vi "meth.PushLVData.vi"(0 "class.GLue in":refnum<class "class.GLue.lvclass">, 7 "variant in":variant, 11 "error in (no error)":errorcluster) -> (4 "class.GLue out":refnum<class "class.GLue.lvclass">, 8 "NumPushed":i32, 15 "error out":errorcluster)   [LabVIEW 2014, in "GLue.lvlib" / "class.GLue.lvclass"]
uses:
  class.GLue.lvclass
  class.GLue.lvclass/class.GLue.ctl
  vi.HeaderFromTD.vi
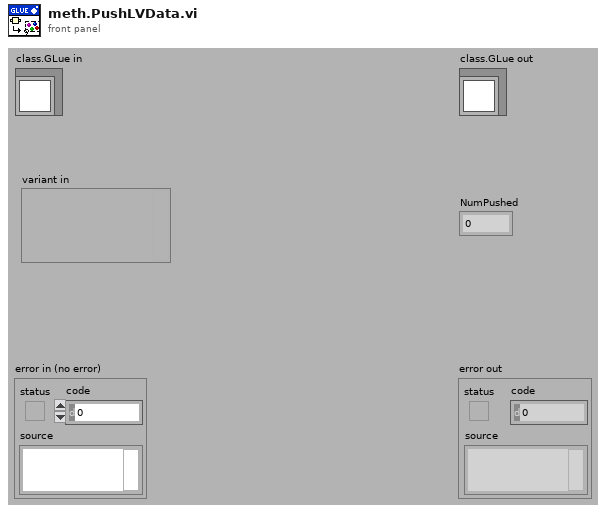
[diagram p1: front panel]
types:
  T1 = enum8{"<Null>", "I8", "I16", "I32", "I64", "U8", "U16", "U32", "U64", "SGL", "DBL", "EXT", "CSG", "CDB", "CXT", "0x0F", "0x10", "0x11", "0x12", "0x13", "0x14", "Enum U8", "Enum U16", "Enum U32", "Enum U64", "SGL PQ", "DBL PQ", "EXT PQ", "CSG PQ", "CDB PQ", "CXT PQ", "0x1F", "0x20", "Boolean", "0x22", "0x23", "0x24", "0x25", "0x26", "0x27", "0x28", "0x29", "0x2A", "0x2B", "0x2C", "0x2D", "0x2E", "0x2F", "String", "0x31", "Path", "Pict", "0x34", "0x35", "0x36", "DAQ", "0x38", "0x39", "0x3A", "0x3B", "0x3C", "0x3D", "0x3E", "0x3F", "Array", "0x41", "0x42", "0x43", "0x44", "0x45", "0x46", "0x47", "0x48", "0x49", "0x4A", "0x4B", "0x4C", "0x4D", "0x4E", "0x4F", "Cluster", "0x51", "0x52", "Variant", "Waveform", "0x55", "0x56", "0x57", "0x58", "0x59", "0x5A", "0x5B", "0x5C", "0x5D", "0x5E", "0x5F", "0x60", "0x61", "0x62", "0x63", "0x64", "0x65", "0x66", "0x67", "0x68", "0x69", "0x6A", "0x6B", "0x6C", "0x6D", "0x6E", "0x6F", "Refnum"}
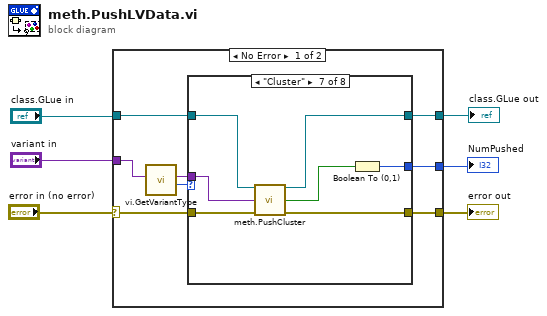
[diagram p0: block diagram]
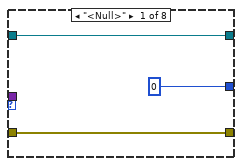
[diagram p2: hidden frame]
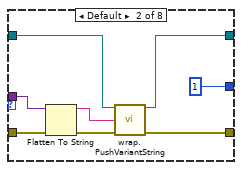
[diagram p3: hidden frame]
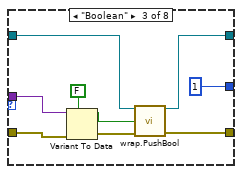
[diagram p4: hidden frame]
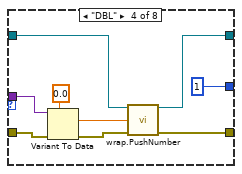
[diagram p5: hidden frame]
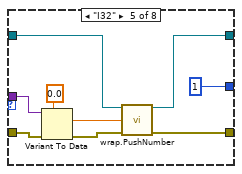
[diagram p6: hidden frame]
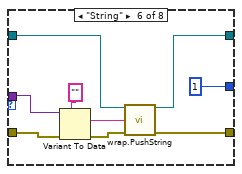
[diagram p7: hidden frame]
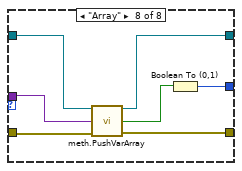
[diagram p8: hidden frame]
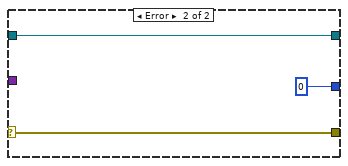
[diagram p9: hidden frame]
diagram:
  n1 = case shown="No Error" "error in (no error)" {
    selector: "error in (no error)" -> [w12 w78]
    tunnel: [w14 w78] -> w5
    tunnel: [w13 w77] -> w2
    tunnel: "class.GLue in" -> [w9 w77]
    tunnel: "variant in" -> [w8 _]
    tunnel: [w7 0] -> w1
    frame No Error {
      n2 = call "vi.GetVariantType.vi"("variant in"=w8) -> ("type"=w10:T1, "variant out"=w11:variant)  [unwired: 9 in]
      n3 = case shown="\"Cluster\"" w10 {
        tunnel: w11 -> [_ w19 w28 w37 w46 w55 w66 w69]
        tunnel: w9 -> [w16 w24 w29 w38 w47 w56 w68 w74]
        tunnel: w12 -> [w17 w22 w31 w40 w49 w58 w67 w75]
        tunnel: [w17 w25 w30 w39 w48 w57 w64 w72] -> w14
        tunnel: [w16 w23 w27 w36 w45 w54 w65 w73] -> w13
        tunnel: [0 1 1 1 1 1 w62 w71] -> w7
        frame "<Null>" {
        }
        frame Default {
          n4 = Flatten To String(anything=w19, error in (no error)=w22) -> (data string=w20:string, error out=w21:errorcluster)  [unwired: 2 in, 1 out]
          n5 = call "wrap.PushVariantString.vi"("class.GLue in"=w24, "VariantString"=w20, "error in (no error)"=w21) -> ("class.GLue out"=w23:refnum<class "class.GLue.lvclass">, "error out"=w25:errorcluster)  [unwired: 11 in]
        }
        frame "Boolean" {
          n6 = Variant To Data(error in=w31, type=FALSE, Variant=w28) -> (data=w34:bool, error out=w33:errorcluster)
          n7 = call "wrap.PushBool.vi"("class.GLue in"=w29, "Boolean"=w34, "error in (no error)"=w33) -> ("class.GLue out"=w27:refnum<class "class.GLue.lvclass">, "error out"=w30:errorcluster)  [unwired: 11 in]
        }
        frame "DBL" {
          n8 = Variant To Data(error in=w40, type=0.0, Variant=w37) -> (data=w41:dbl, error out=w42:errorcluster)
          n9 = call "wrap.PushNumber.vi"("class.GLue in"=w38, "Numeric"=w41, "error in (no error)"=w42) -> ("class.GLue out"=w36:refnum<class "class.GLue.lvclass">, "error out"=w39:errorcluster)  [unwired: 11 in]
        }
        frame "I32" {
          n10 = Variant To Data(error in=w49, type=0.0, Variant=w46) -> (data=w50:dbl, error out=w51:errorcluster)
          n11 = call "wrap.PushNumber.vi"("class.GLue in"=w47, "Numeric"=w50, "error in (no error)"=w51) -> ("class.GLue out"=w45:refnum<class "class.GLue.lvclass">, "error out"=w48:errorcluster)  [unwired: 11 in]
        }
        frame "String" {
          n12 = Variant To Data(error in=w58, type="", Variant=w55) -> (data=w61:string, error out=w60:errorcluster)
          n13 = call "wrap.PushString.vi"("class.GLue in"=w56, "String"=w61, "error in (no error)"=w60) -> ("class.GLue out"=w54:refnum<class "class.GLue.lvclass">, "error out"=w57:errorcluster)  [unwired: 11 in]
        }
        frame "Cluster" {
          n14 = call "meth.PushCluster.vi"("class.GLue in"=w68, "Cluster"=w66, "error in"=w67) -> ("class.GLue out"=w65:refnum<class "class.GLue.lvclass">, "Pushed?"=w63:bool, "error out"=w64:errorcluster)  [unwired: 10 in]
          n15 = Boolean To (0,1)(Boolean=w63) -> (0, 1=w62:i16)
        }
        frame "Array" {
          n16 = call "meth.PushVarArray.vi"("class.GLue in"=w74, "VarArray"=w69, "error in (no error)"=w75) -> ("class.GLue out"=w73:refnum<class "class.GLue.lvclass">, "Pushed?"=w70:bool, "error out"=w72:errorcluster)  [unwired: 10 in]
          n17 = Boolean To (0,1)(Boolean=w70) -> (0, 1=w71:i16)
        }
      }
    }
    frame Error {
    }
  }
  "error out" <- w5
  "class.GLue out" <- w2
  "NumPushed" <- w1
